vi "New Triggered Log.vi"(4 "Posttrigger Samples (-1: Log indefinitely)":i64, 5 "Minimum Buffer Size (1024)":i64=1024, 6 "Pretrigger Samples (0)":i64, 7 "Channel Specifications":T1[](array[typedef]), 8 "error in (no error)":errorcluster, 9 "Stop Trigger":refnum<class "Trigger.lvclass">, 10 "Start Trigger Specification":T2, 11 "Segmented Log Ref":refnum<data-value>) -> (0 "error out":errorcluster, 3 "Triggered Log out":refnum<class "Triggered Log.lvclass">)   [LabVIEW 2015, in "Triggered Log.lvclass"]
doc: "This VI creates a new triggered log instance that operates on the specified segmented log instance. The specified array of channel specifications must match up with the 1D data supplied when logging data to disk.\n\nThe Start Trigger specifies the condition that determines when logging starts. The Retriggerable option determines if the log waits for another start trigger after it has completed logging following the first start trigger. The number of samples specified in Pretrigger Samples determines the number of samples that are buffered while waiting for the start trigger to occur. When the start trigger occurs, any samples in the pretrigger buffer are logged.\n\nThe Stop Trigger specifies the condition that determines when logging stops after it has started. The Posttrigger Samples count specifies how many samples are logged after the stop trigger occurs."
uses:
  Triggered Log.lvclass
  Start Trigger Specification.ctl
  Engine/Classes/Triggers/Trigger/Trigger.lvclass
  Engine/Classes/Logs/Segmented Logs/Segmented Log/Segmented Log.lvclass
  Channel Specification.ctl
  Triggered Log State.ctl
  Triggered Log.lvclass/Triggered Log.ctl
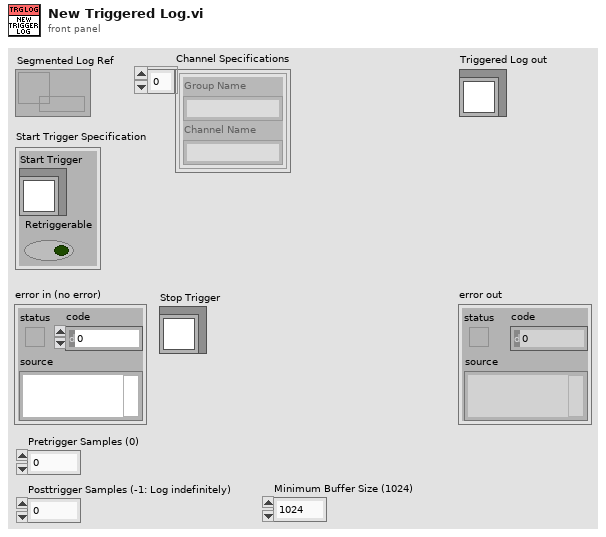
[diagram p1: front panel]
types:
  T1 = typedef "Triggered Log.lvclass/Channel Specification.ctl" = cluster{"Group Name":string, "Channel Name":string}
  T2 = typedef "Triggered Log.lvclass/Start Trigger Specification.ctl" = cluster{"Start Trigger":refnum<class "Trigger.lvclass">, "Retriggerable":bool}
  T3 = typedef "Triggered Log.lvclass/Triggered Log State.ctl" = enum16{"Waiting on Trigger", "Triggered", "Posttrigger", "Complete", "Idle", "Error"}
  T4 = typedef "Triggered Log.lvclass/Buffer Data.ctl" = cluster{"Position":i32, "Length":i32, "Max Length":i32, "Channel Count":i32, "Data":dbl[][], "t0 Array":timestamp[]}
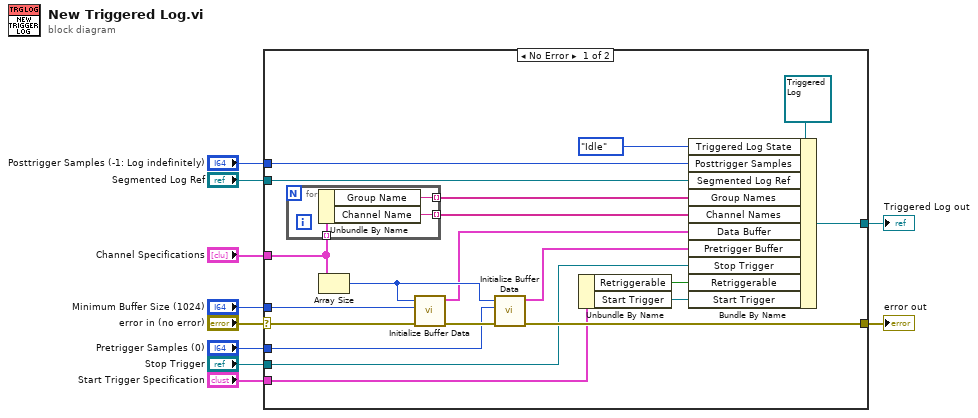
[diagram p0: block diagram]
diagram:
  n1 = case shown="No Error" "error in (no error)" {
    selector: "error in (no error)" -> [w15 w34]
    tunnel: [w30 w34] -> w9
    tunnel: [w28 _] -> w8
    tunnel: "Pretrigger Samples (0)" -> [w14 _]
    tunnel: "Start Trigger Specification" -> [w19 _]
    tunnel: "Segmented Log Ref" -> [w17 _]
    tunnel: "Posttrigger Samples (-1: Log indefinitely)" -> [w27 _]
    tunnel: "Channel Specifications" -> [w20 _]
    tunnel: "Minimum Buffer Size (1024)" -> [w13 _]
    tunnel: "Stop Trigger" -> [w11 _]
    frame No Error {
      n2 = for {
        tunnel: w20 -> [w33] mode=indexing
        tunnel: [w32] -> w23 mode=indexing
        tunnel: [w31] -> w22 mode=indexing
        n3 = Unbundle By Name(w33) -> ("Group Name"=w32:string, "Channel Name"=w31:string)
      }
      n4 = Array Size(array=w20) -> (size(s)=w29:i32)
      n5 = call "Initialize Buffer Data.vi"("error in (no error)"=w15, "Buffer Size"=w13, "Channel Count"=w29) -> ("error out"=w26:errorcluster, "Buffer Data"=w24:T4)  [unwired: 7 in]
      n6 = call "Initialize Buffer Data.vi"("error in (no error)"=w26, "Buffer Size"=w14, "Channel Count"=w29) -> ("error out"=w30:errorcluster, "Buffer Data"=w25:T4)  [unwired: 7 in]
      n7 = Unbundle By Name(w19) -> ("Retriggerable"=w16:bool, "Start Trigger"=w12:refnum<class "Trigger.lvclass">)
      n8 = Bundle By Name(cluster=refnum<class "Triggered Log.lvclass"> refnum ("Triggered Log in"), "Triggered Log State"=Triggered_Log_State."Idle", "Posttrigger Samples"=w27, "Segmented Log Ref"=w17, "Group Names"=w23, "Channel Names"=w22, "Data Buffer"=w24, "Pretrigger Buffer"=w25, "Stop Trigger"=w11, "Retriggerable"=w16, "Start Trigger"=w12) -> (w28:refnum<class "Triggered Log.lvclass">)
    }
    frame Error {
    }
  }
  "error out" <- w9
  "Triggered Log out" <- w8
